vi "SerialVI.vi"() -> ()   [LabVIEW 2017]
uses:
  <vilib>/Instr/_visa.llb/VISA Flush IO Buffer Mask.ctl
  <vilib>/Instr/_visa.llb/VISA Configure Serial Port (Instr).vi
panel:
  out "VISA resource name out":refnum<visa-resource-name>
  in  "stop":bool
  out "state":dbl
  out "message window":string
  out "read buffer":string
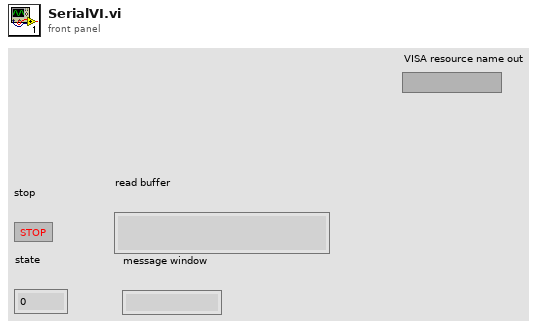
[diagram p1: front panel]
types:
  T1 = typedef "VISA Flush IO Buffer Mask.ctl" = u16
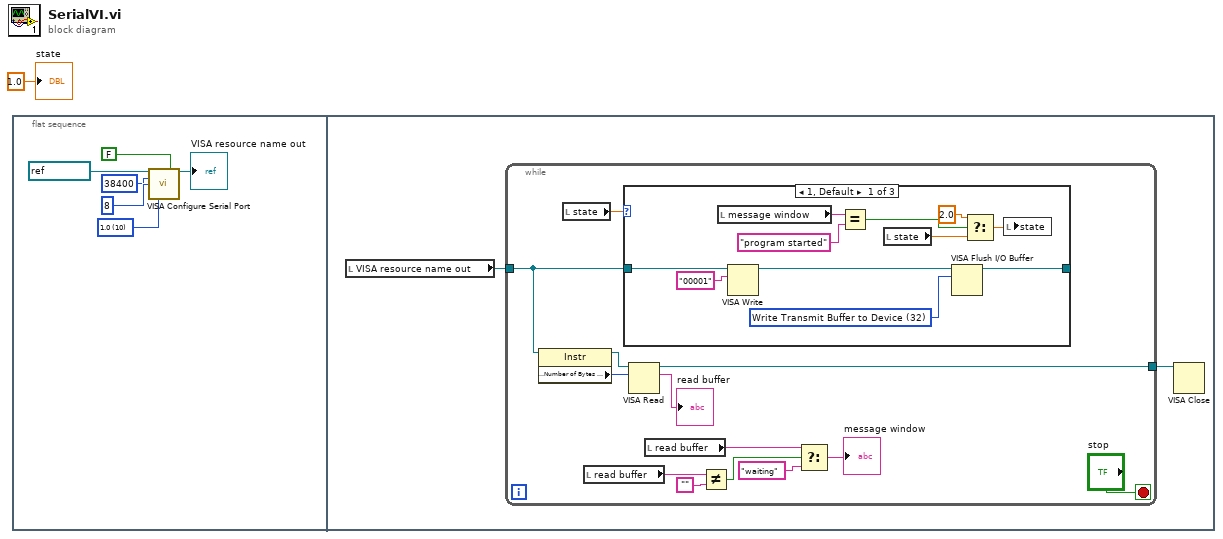
[diagram p0: block diagram]
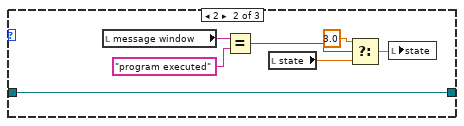
[diagram p2: hidden frame]
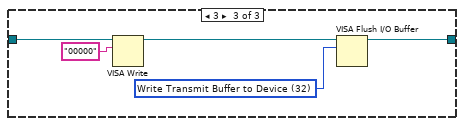
[diagram p3: hidden frame]
diagram:
  n1 = flat-sequence {
    frame #0 {
      w4 = u16 10 items=["1.0"=10, "1.5"=15, "2.0"=20] ("stop bits (10: 1 bit)")
      n2 = call-poly "VISA Configure Serial Port"("VISA resource name"=refnum<visa-resource-name> "COM2", "Enable Termination\nChar (T)"=FALSE ("Enable Termination\nChar (T)"), "baud rate (9600)"=u32 38400, "data bits (8)"=u16 8, "stop bits (10: 1 bit)"=w4) -> ("VISA resource name out"=→"VISA resource name out":refnum<visa-resource-name>)  [unwired: 9 in, 1 out]
    }
    frame #1 {
      n3 = local read "VISA resource name out"() -> (w9:refnum<visa-resource-name>)
      n4 = while {
        tunnel: w9 -> [w22]
        tunnel: [w21] -> w8
        stop <- "stop" stop-if-true
        n5 = property class="Instr"(reference=w22) -> (reference out=w20:refnum<visa-resource-name>, "Serial Settings:Number of Bytes at Serial Port"=w18:u32)  [unwired: 1 in, 1 out]
        n6 = local read "state"() -> (w10:dbl)
        n7 = local read "read buffer"() -> (w13:string)
        n8 = case shown="1, Default" w10 {
          tunnel: [w31 w34 w43] -> _
          tunnel: w22 -> [w33 w34 w45]
          frame 1, Default {
            w30 = T1 32 items=["Flush Receive Buffer"=16, "Write Transmit Buffer to Device"=32, "Flush Receive Buffer (No I/O)"=64, "Flush Transmit Buffer"=128] ("Mask")
            n9 = local read "message window"() -> (w28:string)
            n10 = VISA Write(VISA resource name=w33, write buffer="00001") -> (VISA resource name out=w32:refnum<visa-resource-name>)  [unwired: 1 in, 2 out]
            n11 = Equal?(x=w28, y="program started") -> (x = y?=w24:bool)
            n12 = local read "state"() -> (w23:dbl)
            n13 = VISA Flush I/O Buffer(VISA resource name=w32, mask (16)=w30) -> (VISA resource name out=w31:refnum<visa-resource-name>)  [unwired: 1 in, 1 out]
            n14 = Select(t=2.0, s=w24, f=w23) -> (s? t:f=w25:dbl)
            n15 = local write "state"(w25) -> ()
          }
          frame 2 {
            n16 = local read "message window"() -> (w40:string)
            n17 = Equal?(x=w40, y="program executed") -> (x = y?=w36:bool)
            n18 = local read "state"() -> (w35:dbl)
            n19 = Select(t=3.0, s=w36, f=w35) -> (s? t:f=w37:dbl)
            n20 = local write "state"(w37) -> ()
          }
          frame 3 {
            w42 = T1 32 items=["Flush Receive Buffer"=16, "Write Transmit Buffer to Device"=32, "Flush Receive Buffer (No I/O)"=64, "Flush Transmit Buffer"=128] ("Mask")
            n21 = VISA Write(VISA resource name=w45, write buffer="00000") -> (VISA resource name out=w44:refnum<visa-resource-name>)  [unwired: 1 in, 2 out]
            n22 = VISA Flush I/O Buffer(VISA resource name=w44, mask (16)=w42) -> (VISA resource name out=w43:refnum<visa-resource-name>)  [unwired: 1 in, 1 out]
          }
        }
        n23 = VISA Read(VISA resource name=w20, byte count=w18) -> (VISA resource name out=w21:refnum<visa-resource-name>, read buffer=→"read buffer":string)  [unwired: 1 in, 2 out]
        n24 = local read "read buffer"() -> (w15:string)
        n25 = Not Equal?(x=w13, y="") -> (x != y?=w16:bool)
        n26 = Select(t=w15, s=w16, f="waiting") -> (s? t:f=→"message window":string)
      }
      n27 = VISA Close(VISA resource name=w8) -> ()  [unwired: 1 in, 1 out]
    }
  }
  "state" <- 1.0 ("state")
